vi "DS写属性数据.vi"() -> ()   [LabVIEW 2010]
uses:
  <vilib>/Analysis/NI_AALBase.lvlib
panel:
  in  "停止":bool
  out "波形图":dbl[](graph)
  in  "幅值":dbl(slide)=1.0 scale=0.0..10.0
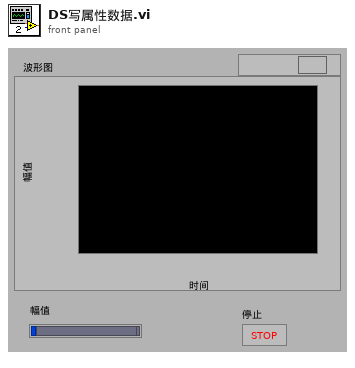
[diagram p1: front panel]
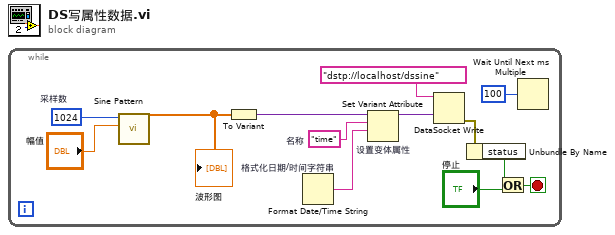
[diagram p0: block diagram]
diagram:
  n1 = while {
    stop <- w5 stop-if-true
    w7 = 1024  # 采样数
    w9 = "time"  # 名称
    n2 = call <vilib>:"Sine Pattern.vi"("amplitude"="幅值", "samples"=w7) -> ("Sinusoidal Pattern"=w12:dbl[])  [unwired: 2 in, 1 out]
    "波形图" <- w12
    n3 = To Variant(anything=w12) -> (Variant=w10:variant)
    n4 = Format Date/Time String "格式化日期/时间字符串"() -> (date/time string=w8:string)  [unwired: 3 in]
    n5 = Set Variant Attribute "设置变体属性"(Variant=w10, name=w9, value=w8) -> (Variant out=w11:variant)  [unwired: 1 in, 2 out]
    n6 = DataSocket Write(10:w11, 11:"dstp://localhost/dssine" ("URL")) -> (0:w4:errorcluster)  [unwired: 2 in, 2 out]
    n7 = Unbundle By Name(w4) -> ("status"=w3:bool)
    n8 = Or(x=w3, y="停止") -> (x .or. y?=w5:bool)
    n9 = Wait Until Next ms Multiple(millisecond multiple=u32 100) -> ()  [unwired: 1 out]
  }
